vi "Get Filenames in Directory.vi"(8 "error in":errorcluster, 11 "directory path":path=path "C:/ATS Development/Code/MyCalc") -> (0 "error out":errorcluster, 2 "filepath array":path[](array[path]))   [LabVIEW 2010]
doc: "This function returns a list of filenames (array of filepaths) in a directory."
panel:
  out "path count":i32=-1
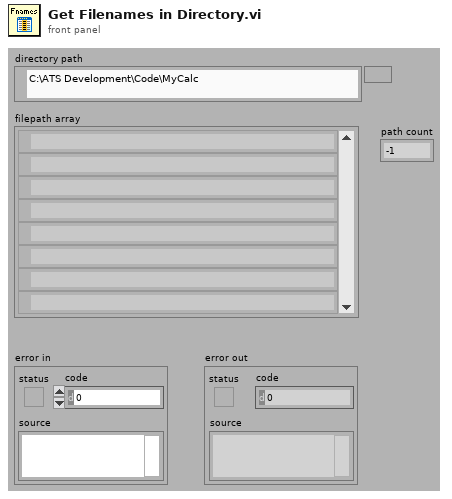
[diagram p1: front panel]
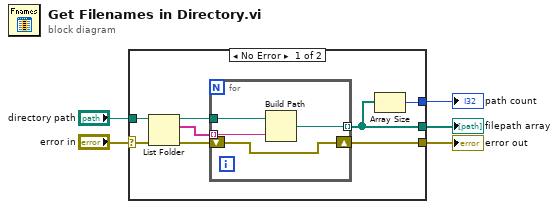
[diagram p0: block diagram]
diagram:
  n1 = case shown="No Error" "error in" {
    selector: "error in" -> [w13 w18]
    tunnel: "directory path" -> [w12 _]
    tunnel: [w8 w18] -> w4
    tunnel: [w7 _] -> w2
    tunnel: [w6 _] -> w1
    frame No Error {
      n2 = List Folder(path=w12, error in=w13) -> (path out=w11:path, filenames=w9:string[], error out=w10:errorcluster)  [unwired: 2 in, 1 out]
      n3 = for {
        tunnel: w11 -> [w17]
        shift-right: [w15] -> w8
        shift-left: w10 -> [w15]
        tunnel: w9 -> [w16] mode=indexing
        tunnel: [w14] -> w7 mode=indexing
        n4 = Build Path(base path=w17, name or relative path=w16) -> (appended path=w14:path)
      }
      n5 = Array Size(array=w7) -> (size(s)=w6:i32)
    }
    frame Error {
    }
  }
  "error out" <- w4
  "filepath array" <- w2
  "path count" <- w1
